vi "Stop Core.vi"(10 "final error code":i32, 11 "Ex Nested in":refnum<class "Instrument Actor.lvclass">) -> (3 "Ex Nested out":refnum<class "Instrument Actor.lvclass">)   [LabVIEW 2016, in "Instrument Actor.lvclass"]
doc: "(<B>Filename</B>: Actor Framework.lvlib:Actor.lvclass:Stop Core.vi)\n\nDefines what the actor does before it stops. Use the <B>final error code</B> input to determine whether the actor shut down in response to an error.\n\nBy default, this method does nothing. A descendant class may override it to define behavior, such as shutting down any processes the actor initiated in its override of the Actor Core method."
uses:
  Instrument Actor.lvclass
  G:/sw_repo/For Builds/Reusable/SuperActor/SuperActor.lvclass
  SuperActor/SuperActor.lvclass/SuperActor.ctl
  Instrument Actor.lvclass/Instrument Actor.ctl
  Instrument.lvclass/Instrument.ctl
  SuperActor/Read Log Session.vi
  SuperActor/Read ID.vi
  Read Instr.vi
  Read CMD.vi
  Command/Command.lvclass
  Instrument.lvclass
  Session APIs/_Session Fwk/Session - Root.lvclass
  SuperActor/SuperActor.lvclass
  Session APIs/Session Log/System Log.lvclass
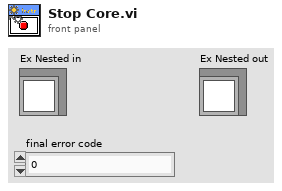
[diagram p1: front panel]
types:
  T1 = typedef "Session - Root.lvclass/Session Handle.ctl" = refnum<data-value>
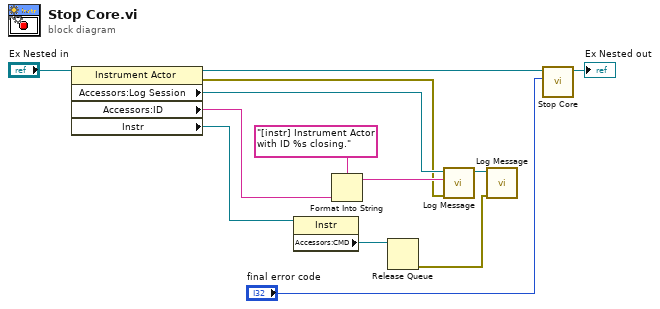
[diagram p0: block diagram]
diagram:
  n1 = property class="Instrument Actor"(reference="Ex Nested in") -> (reference out=w5:refnum<class "Instrument Actor.lvclass">, error out=w6:errorcluster, "Accessors:Log Session"=w10:T1, "Accessors:ID"=w8:string, "Instr"=w4:refnum<class "Instrument.lvclass">)  [unwired: 1 in]
  n2 = property class="Instr"(reference=w4) -> ("Accessors:CMD"=w3:refnum<queue>)  [unwired: 1 in, 2 out]
  n3 = Format Into String(format string="[instr] Instrument Actor with ID %s closing.", w8) -> (resulting string=w7:string)  [unwired: 2 in, 1 out]
  n4 = Release Queue(queue=w3) -> (error out=w1:errorcluster)  [unwired: 2 in, 2 out]
  n5 = call "Log Message.vi"("error in"=w6, "MSG In"=w7, "session in"=w10) -> ("session out"=w2:T1)  [unwired: 7 in, 1 out]
  n6 = call "Log Message.vi"("error in"=w1, "session in"=w2) -> ()  [unwired: 8 in, 2 out]
  n7 = call-parent "Stop Core.vi"("final error code"="final error code", "Ex Nested in"=w5) -> ("Ex Nested out"=→"Ex Nested out":refnum<class "Instrument Actor.lvclass">)  [unwired: 9 in]
